vi "Cluster (Structure).vi"() -> ()   [LabVIEW 2020]
panel:
  out "String 2":string
  out "Boolean 2":bool
  out "Numeric 2":dbl
  out "output cluster":T1
  out "String":string
  out "Boolean":bool
  out "Numeric":dbl
  in  "Cluster":T1
  # "Cluster (Structure)"
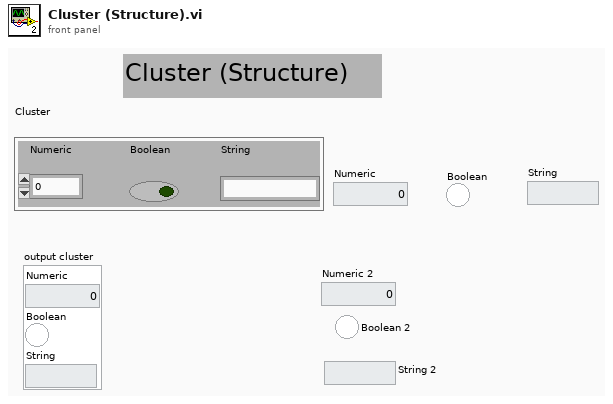
[diagram p1: front panel]
types:
  T1 = cluster{"Numeric":dbl, "Boolean":bool, "String":string}
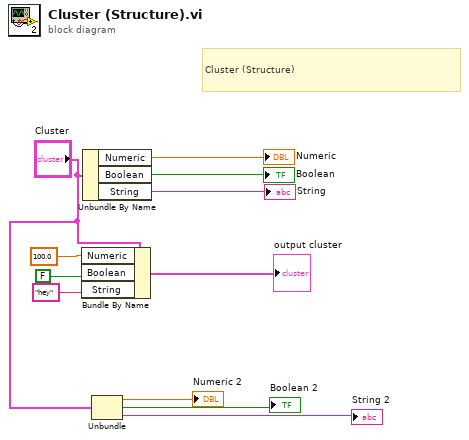
[diagram p0: block diagram]
diagram:
  # "Cluster (Structure)"
  n1 = Bundle By Name "Bundle By Name"(cluster="Cluster", "Numeric"=100.0, "Boolean"=FALSE, "String"="hey") -> (→"output cluster":T1)
  n2 = Unbundle By Name "Unbundle By Name"("Cluster") -> ("Numeric"=→"Numeric":dbl, "Boolean"=→"Boolean":bool, "String"=→"String":string)
  n3 = Unbundle "Unbundle"("Cluster") -> ("Numeric"=→"Numeric 2":dbl, "Boolean"=→"Boolean 2":bool, "String"=→"String 2":string)
